vi "Core Write U8 FIFO.vi"(7 "Includes Header":bool, 8 "error in (no error)":errorcluster, 10 "U8 in":u8[](array[numeric]), 11 "CIFFIFO in":refnum<class "CIF_CIPC_Fifo_U8.lvclass">) -> (0 "error out":errorcluster, 2 "U8 out":u8[](array[numeric]), 3 "CIFFIFO out":refnum<class "CIF_CIPC_Fifo_U8.lvclass">)   [LabVIEW 2021, in "CIF_CIPC_Fifo_U8.lvclass"]
uses:
  CIF_CIPC_Fifo_U8.lvclass
  D:/dev/Packages/CIF_Channels_Core/src/CIFChannels/CIFChannels.lvclass
  D:/dev/Packages/CIF_Channels_Core/src/CIPC_Channels/CIF_CIPC_Chan/CIF_CIPC_Chn.lvclass
  CIFChannels/CIFChannels.lvclass/CIFChannels.ctl
  CIF_CIPC_Chan/CIF_CIPC_Chn.lvclass/CIF_CIPC_Chn.ctl
  <vilib>/CIF Foundation/CIF CIPC/TypeDefs/Partial Write Configuration.ctl
  <vilib>/CIF Foundation/CIF Utilities/Statistics/I64/Stats_I64_CIF_U.lvclass/Stats_I64_CIF_U.ctl
  1bad10da-a98b-49ee-b03a-18b497e396df.vi
  70f860b1-5d4a-43dc-b0c2-c9446e8447f7.vi
  40f8d1bb-2a62-444a-8ee6-d4d6c496dc12.vi
  CIFChannels/Accessors/Read FIFO Header.vi
  <vilib>/CIF Foundation/CIF Utilities/Statistics/I64/X1 minus X0.vi
  <vilib>/CIF Foundation/CIF Utilities/Time/System Time/Get System Time.vi
  <vilib>/CIF Foundation/CIF CIPC/SubVIs/Check Error.vi
  <vilib>/CIF Foundation/CIF CIPC/SubVIs/Notify Of New Write.vi
  <vilib>/CIF Foundation/CIF CIPC/SubVIs/Get dll Path.vi
  <vilib>/CIF Foundation/CIF CIPC/SubVIs/Get Element Write Position.vi
  <vilib>/CIF Foundation/CIF Utilities/Statistics/I64/X1 minus X0.vi/dfabcf33-0dbc-4041-80a5-3dc0c86d2989.vi
  <vilib>/CIF Foundation/CIF Utilities/Time/System Time/LabVIEW Time to TAI Time.vi
  <vilib>/CIF Foundation/CIF Utilities/Statistics/I64/X1 minus X0.vi/dfabcf33-0dbc-4041-80a5-3dc0c86d2989.vi/9eb60a9a-770f-4d2d-8b3f-8465c267ecc9.vi
  <vilib>/Utility/error.llb/Trim Whitespace.vi
  <vilib>/Utility/error.llb/Error Cluster From Error Code.vi
  CIF_CIPC_Fifo_U8.lvclass/CIF_CIPC_Fifo_U8.ctl
  CIFChannels/CIFChannels.lvclass
  CIF_CIPC_Chan/CIF_CIPC_Chn.lvclass
  <vilib>/CIF Foundation/CIF CIPC/CIF_NI_CIPC.lvlib
  ChannelCommon/ChannelCommon.lvlib
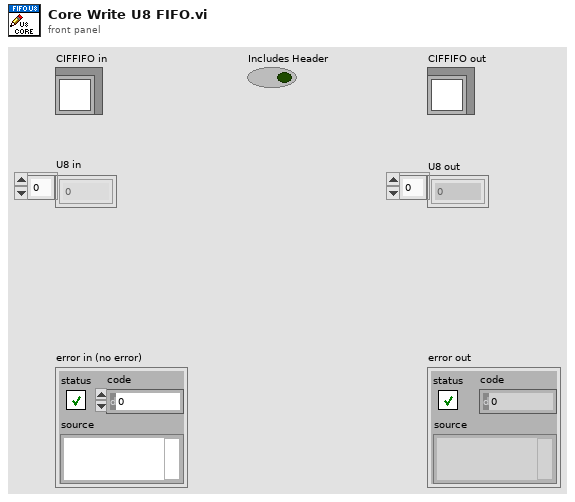
[diagram p1: front panel]
types:
  T1 = typedef "CIF_NI_CIPC.lvlib/Partial Write Configuration.ctl" = cluster{"Start Offset (bytes)":u32, "Total Length (bytes)":u32, "Last Write":bool, "Get Write Position":bool, "Notify Readers":bool}
  T2 = typedef "ChannelCommon.lvlib/FIFO Header.ctl" = cluster{"Length":u64, "T0":i64, "T_Out":i64, "T_Tx":i64, "Ctr":u64, "ClockID":u8}
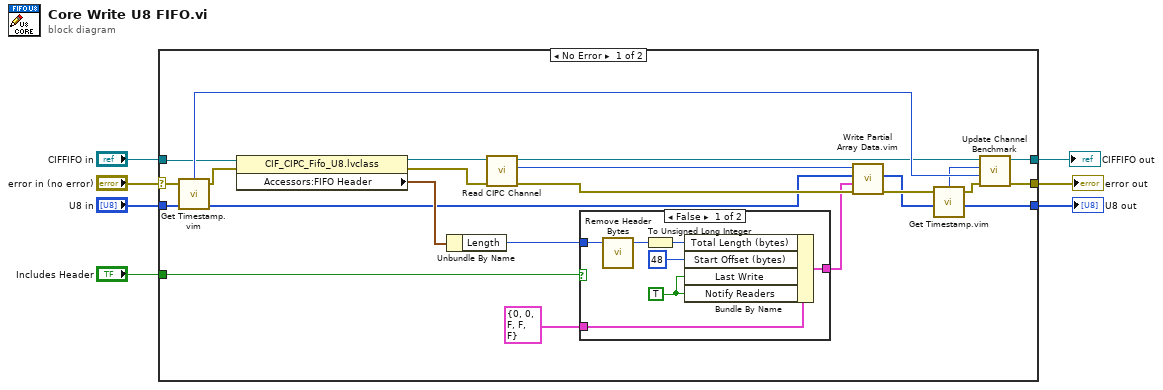
[diagram p0: block diagram]
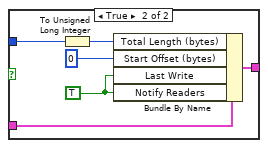
[diagram p2: hidden frame]
diagram:
  n1 = case shown="No Error" "error in (no error)" {
    selector: "error in (no error)" -> [w22 w44]
    tunnel: [w27 w44] -> w6
    tunnel: [w26 w43] -> w2
    tunnel: "CIFFIFO in" -> [w23 w43]
    tunnel: "U8 in" -> [w13 w42]
    tunnel: [w12 w42] -> w4
    tunnel: "Includes Header" -> [w9 _]
    frame No Error {
      n2 = call "Get Timestamp.vim"("Anything in"=w22) -> ("Time (ns)"=w25:i64, "Anything out"=w21:errorcluster)  [unwired: 2 in]
      n3 = property class="CIF_CIPC_Fifo_U8.lvclass"(reference=w23, error in=w21) -> (reference out=w18:refnum<class "CIF_CIPC_Fifo_U8.lvclass">, error out=w19:errorcluster, "Accessors:FIFO Header"=w28:T2)
      n4 = Unbundle By Name(w28) -> ("Length"=w8:u64)
      n5 = call "Read CIPC Channel.vi"("error in (no error)"=w19, "CIFTag in"=w18) -> ("error out"=w15:errorcluster, "CIPC Channel"=w16:u64, "CIFTag out"=w17:refnum<class "CIF_CIPC_Fifo_U8.lvclass">)  [unwired: 7 in]
      n6 = case shown="False" w9 {
        tunnel: T1 {"Start Offset (bytes)"=0, "Total Length (bytes)"=0, "Last Write"=FALSE, "Get Write Position"=FALSE, "Notify Readers"=FALSE} ("Partial Write Configuration") -> [w35 w41]
        tunnel: [w33 w39] -> w10
        tunnel: w8 -> [w31 w37]
        frame False {
          w34 = TRUE ("Last Write")
          n7 = call "Remove Header Bytes.vi"("Bytes/Msg with header"=w31) -> ("Bytes/Msg without header"=w30:u64)  [unwired: 3 in]
          n8 = To Unsigned Long Integer(number=w30) -> (unsigned 32bit integer=w29:u32)
          n9 = Bundle By Name(cluster=w35, "Total Length (bytes)"=w29, "Start Offset (bytes)"=u32 48 ("y"), "Last Write"=w34, "Notify Readers"=w34) -> (w33:T1)
        }
        frame True {
          w40 = TRUE ("Last Write")
          n10 = To Unsigned Long Integer(number=w37) -> (unsigned 32bit integer=w36:u32)
          n11 = Bundle By Name(cluster=w41, "Total Length (bytes)"=w36, "Start Offset (bytes)"=u32 0 ("y"), "Last Write"=w40, "Notify Readers"=w40) -> (w39:T1)
        }
      }
      n12 = call "Write Partial Array Data.vim"("error in (no error)"=w15, "Partial Write Configuration"=w10, "Data in"=w13, "CIPC Reference in"=w16) -> ("error out"=w14:errorcluster, "Data out"=w12:u8[])  [unwired: 4 in, 2 out]
      n13 = call "Get Timestamp.vim"("Anything in"=w14) -> ("Time (ns)"=w24:i64, "Anything out"=w20:errorcluster)  [unwired: 2 in]
      n14 = call "Update Channel Benchmark.vi"("error in (no error)"=w20, "X0"=w25, "X1"=w24, "CIFChannels in"=w17) -> ("error out"=w27:errorcluster, "CIFChannels out"=w26:refnum<class "CIF_CIPC_Fifo_U8.lvclass">)  [unwired: 6 in]
    }
    frame Error {
    }
  }
  "error out" <- w6
  "U8 out" <- w4
  "CIFFIFO out" <- w2
